vi "3.4.vi"() -> ()   [LabVIEW 2017]
panel:
  in  "字符串 2":string
  out "长度":dbl
  out "连接后":string
  in  "数值":dbl
  in  "字符串":string
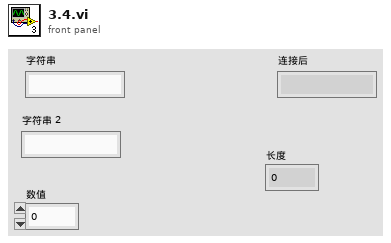
[diagram p1: front panel]
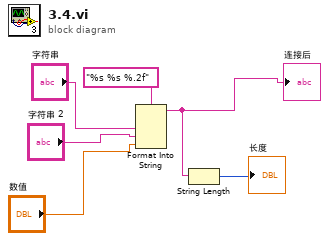
[diagram p0: block diagram]
diagram:
  n1 = Format Into String(format string="%s %s %.2f" ("格式字符串"), "字符串", "字符串 2", "数值") -> (resulting string=w2:string)  [unwired: 2 in, 1 out]
  "连接后" <- w2
  n2 = String Length(string=w2) -> (length=→"长度":i32)
